vi "Post Update.vi"(8 "error in (no error)":errorcluster, 11 "Dual Fan in":refnum<class "Dual Fan.lvclass">) -> (0 "error out":errorcluster, 3 "Dual Fan out":refnum<class "Dual Fan.lvclass">)   [LabVIEW 2012, in "Dual Fan.lvlib" / "Dual Fan.lvclass"]
uses:
  Dual Fan.lvclass
  <vilib>/ActorFramework/Actor/Actor.lvclass/Actor.ctl
  Dual Fan.lvclass/Dual Fan.ctl
  Cooler/Update Fan Status Msg/Update Fan Status Msg.lvclass/Update Fan Status Msg.ctl
  <vilib>/ActorFramework/Message Enqueuer/Message Enqueuer.lvclass/Message Enqueuer.ctl
  <vilib>/ActorFramework/Message Enqueuer/Enqueue.vi
  <vilib>/ActorFramework/Message Priority Queue/Priority Enqueue.vi
  Cooler/Update Fan Status Msg/Update Fan Status Msg.lvclass
  <vilib>/ActorFramework/Actor/Actor.lvclass
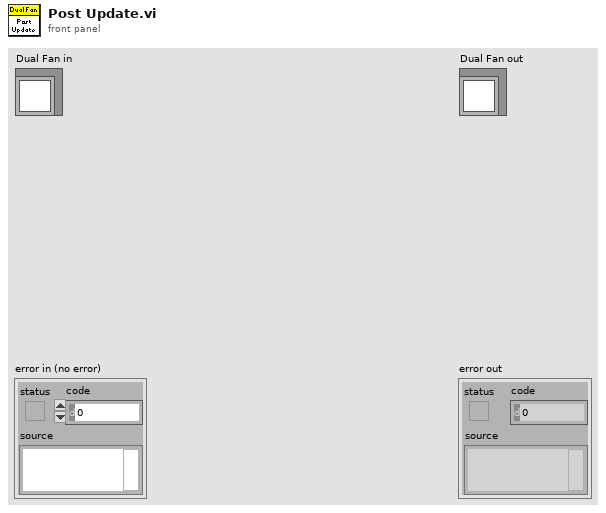
[diagram p1: front panel]
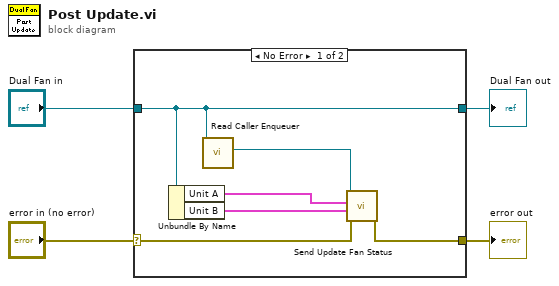
[diagram p0: block diagram]
diagram:
  n1 = case shown="No Error" "error in (no error)" {
    selector: "error in (no error)" -> [w6 w12]
    tunnel: [w5 w12] -> w3
    tunnel: [w10 w11] -> w1
    tunnel: "Dual Fan in" -> [w10 w11]
    frame No Error {
      n2 = Unbundle By Name(w10) -> ("Unit A"=w8:cluster{"State":bool, "Fault":bool}, "Unit B"=w9:cluster{"State":bool, "Fault":bool})
      n3 = call <vilib>:"Read Caller Enqueuer.vi"("Actor"=w10) -> ("Caller Enqueuer"=w7:refnum<class "Message Enqueuer.lvclass">)  [unwired: 10 in]
      n4 = call "Send Update Fan Status.vi"("error in (no error)"=w6, "Fan B"=w9, "Fan A"=w8, "enqueuer"=w7) -> ("error out"=w5:errorcluster)  [unwired: 7 in]
    }
    frame Error {
    }
  }
  "error out" <- w3
  "Dual Fan out" <- w1
